vi "Scope1.vi"(2 "错误输入":errorcluster caption="错误输出") -> (0 "错误输出":errorcluster)   [LabVIEW 2012]
uses:
  Program Files (x86)/National Instruments/LabVIEW 2018/instr.lib/Tektronix DPO MSO 2000 4000 Series/Tektronix DPO MSO 2000 4000 Series.lvlib
panel:
  out "Busy":bool
  in  "电压范围":u64(ring)=10 items=["1 V"=1000000, "100mv"=100000, "10mv"=10000, "1mv"=1000, "100uv"=100, "10uv"=10]
  in  "时间范围":u64(ring)=100000 items=["100ms"=1000000000, "10ms"=100000000, "1ms"=10000000, "100us"=1000000, "10us"=100000, "1us"=10000, "100ns"=1000, "10ns"=100, "1ns"=10, "100ps"=1]
  in  "Channel":T1(ring)
  in  "停止":bool
  in  "开始测量":bool
  in  "更改参数":bool
  out "示波器通信":bool caption="通信正常"
  out "重频":dbl format="%.2f"
  out "脉宽":dbl format="%.2f"
  out "时间波形":waveform(dbl)(graph)
  # "时间波形"
  # "脉冲宽度"
  # "ns"
  # "重复频率"
  # "hz"
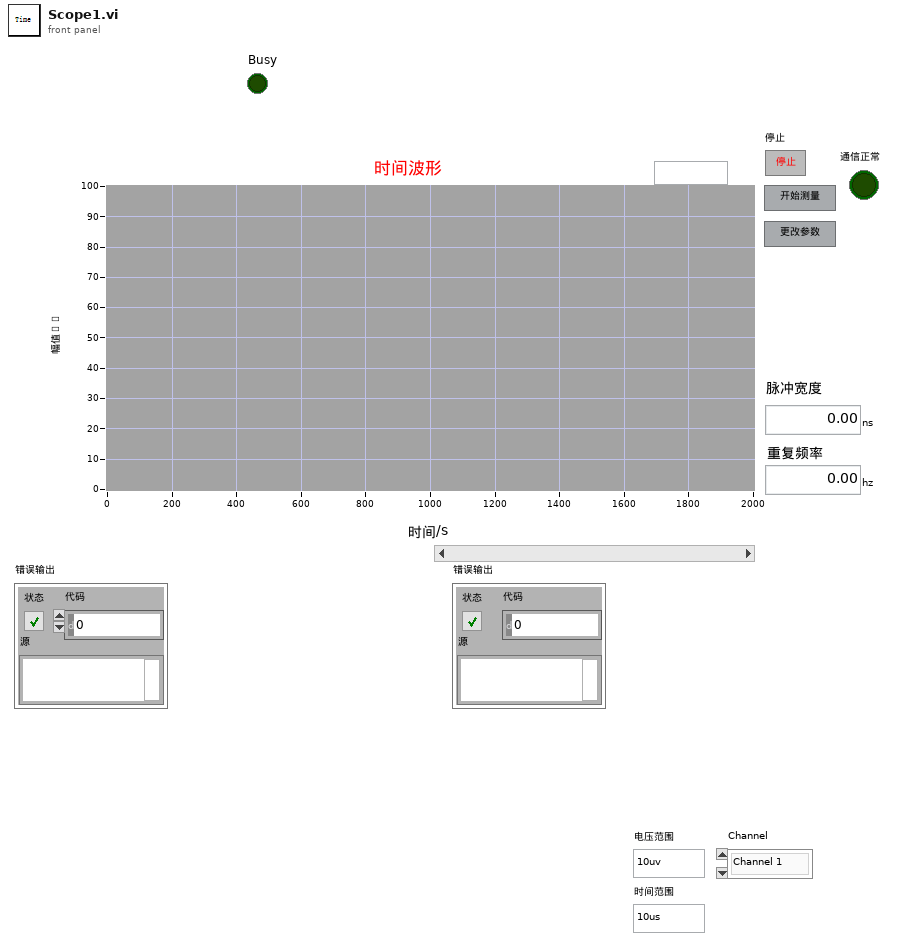
[diagram p1: front panel]
types:
  T1 = enum16{"Channel 1", "Channel 2", "Channel 3", "Channel 4"}
  T2 = typedef "IMAQ Image.ctl" = refnum<image>
  T3 = cluster{"示波器":cluster{"Channel (0:Channel 1)":enum16{"Channel 1", "Channel 2", "Channel 3", "Channel 4"}, "电压范围":dbl, "触发电压":dbl, "时间范围":dbl, " 示波器VISA":refnum<visa-resource-name>}, "光谱仪":cluster{"Channel (0:Channel 1)":enum16{"Channel 1", "Channel 2", "Channel 3", "Channel 4"}, "电压范围":u64, "触发电压":u64, "时间范围":u64}, " 相机1":cluster{"曝光时间":i32, "模拟增益":i32, "控制套接字":i32, "IP 地址":string, " 采集套接字":i32, "  版本号":i32, "ImageData":T2, "  增益最大":i32, "  增益最小":i32, " 曝光最大":i32, " 曝光最小":i32, " 帧速":i32, " 同步切换":i32, "  曝光缩放":i32}, " 偏振仪":cluster{"波长范围":enum16{"可见光", "近红外"}, "电压范围":u64, "触发电压":u64, "时间范围":u64}, " 功率计":cluster{"通道":enum16{"Channel 1", "Channel 2"}, "工作波长":u64, "单位":u64, "时间范围":u64}, "能量计":cluster{"通道":enum16{"Channel 1", "Channel 2"}, "工作波长":u64, "单位":u64, "时间范围":u64}, "电机":cluster{"Channel (0:Channel 1)":enum16{"Channel 1", "Channel 2", "Channel 3", "Channel 4"}, "电压范围":u64, "触发电压":u64, "时间范围":u64}}
  T4 = cluster{"Channel (0:Channel 1)":enum16{"Channel 1", "Channel 2", "Channel 3", "Channel 4"}, "电压范围":dbl, "触发电压":dbl, "时间范围":dbl, " 示波器VISA":refnum<visa-resource-name>}
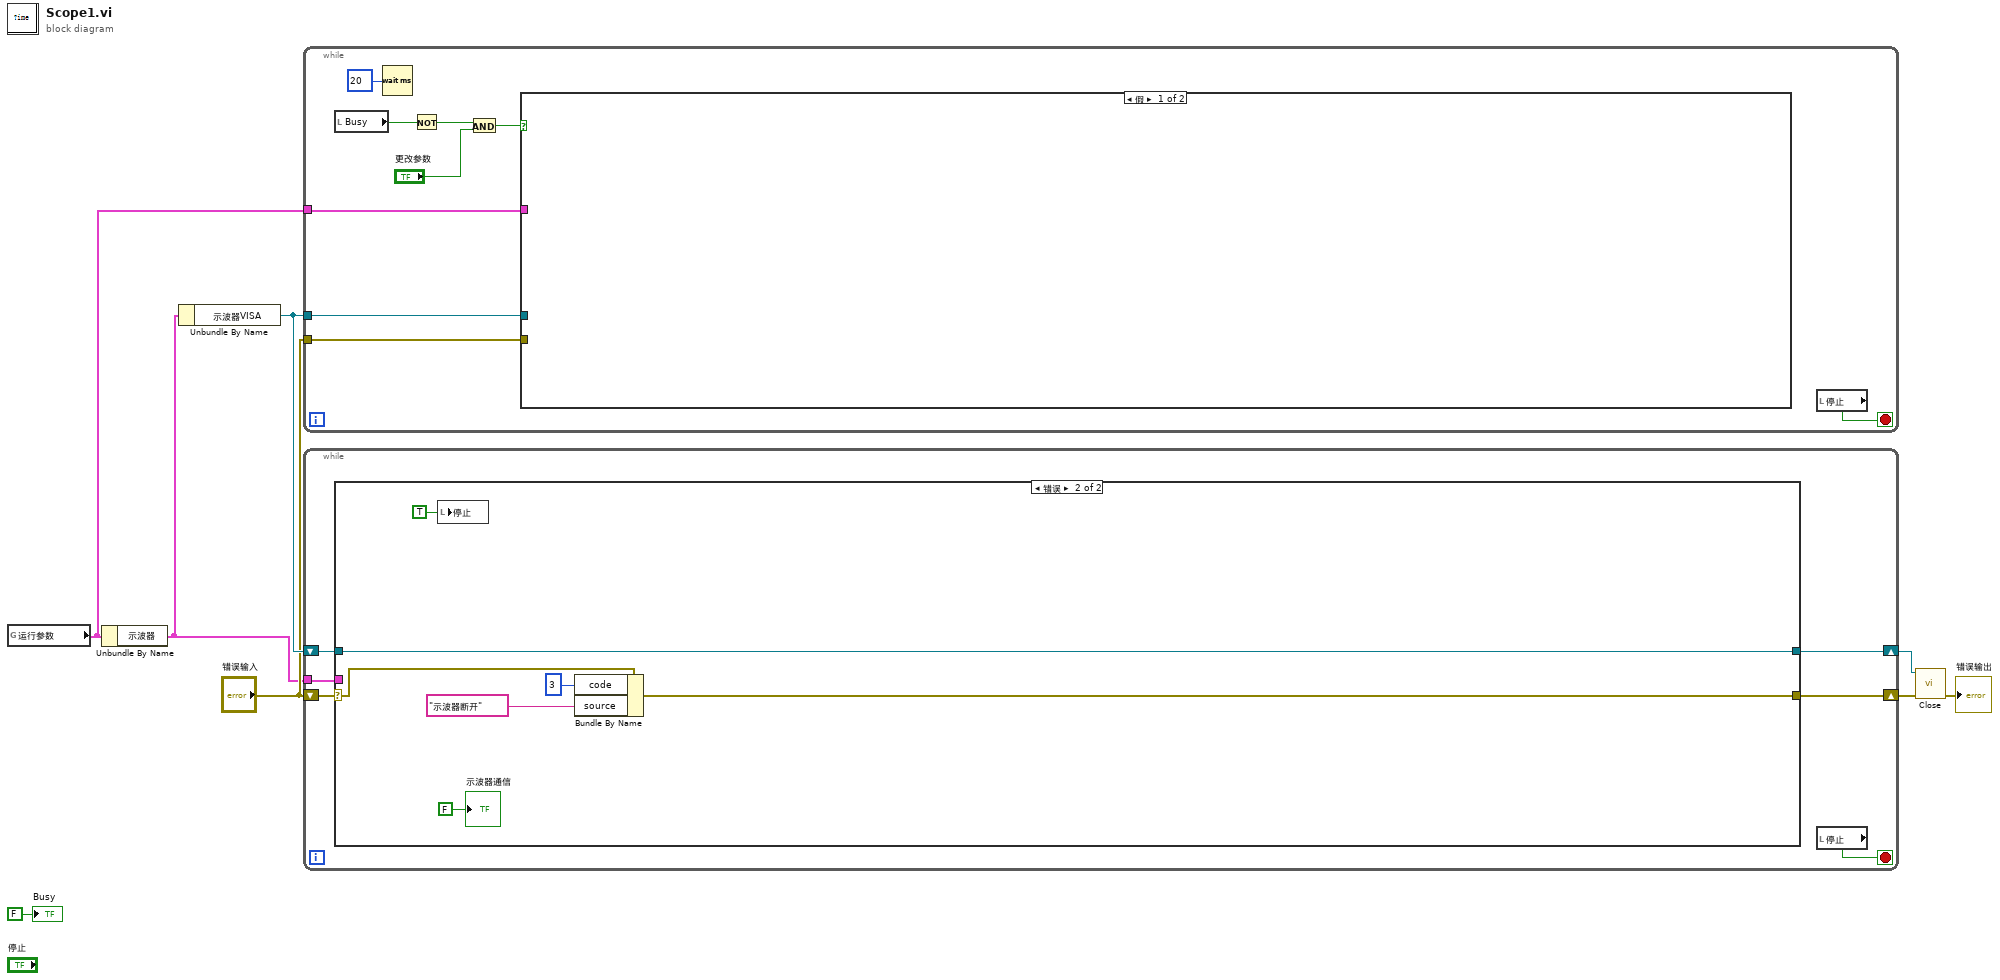
[diagram p0: block diagram]
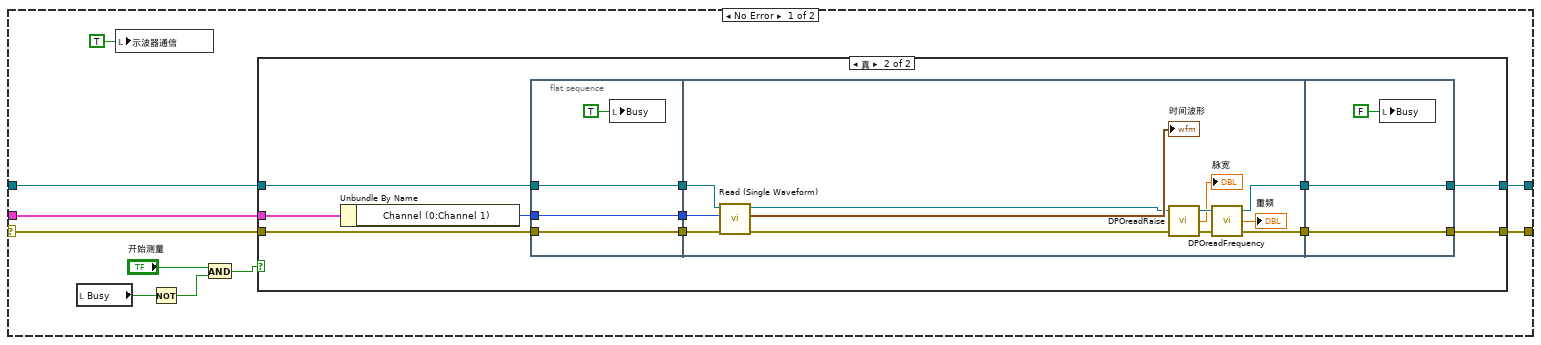
[diagram p2: hidden frame]
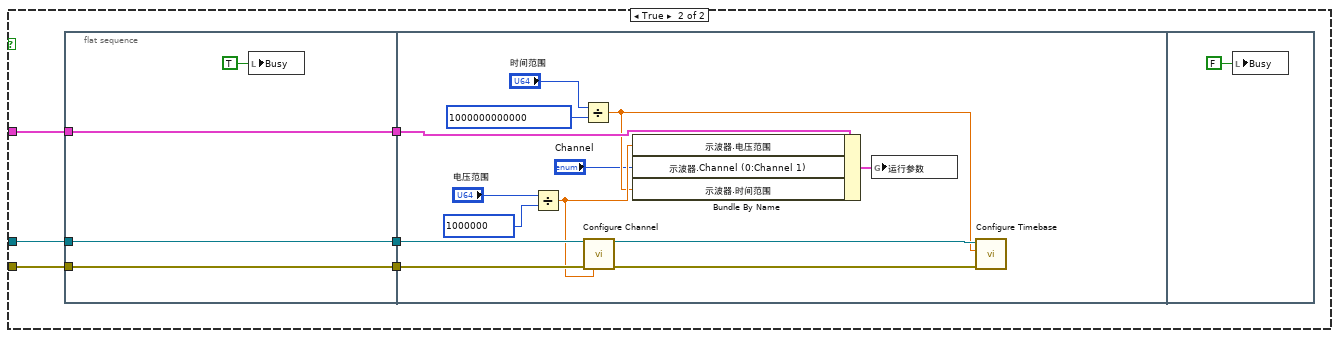
[diagram p4: hidden frame]
diagram:
  n1 = global read "参数.vi" "运行参数"() -> (w4:T3)
  n2 = Unbundle By Name(w4) -> ("示波器"=w1:T4)
  n3 = Unbundle By Name(w1) -> ("示波器VISA"=w5:refnum<visa-resource-name>)
  n4 = while {
    tunnel: w5 -> [w16]
    tunnel: w4 -> [w15]
    tunnel: "错误输入" -> [w14]
    stop <- w17 stop-if-true
    n5 = local read "Busy"() -> (w13:bool)
    n6 = Wait (ms)(milliseconds to wait=u32 20 ("等待时间（毫秒）")) -> ()  [unwired: 1 out]
    n7 = Not(x=w13) -> (.not. x?=w12:bool)
    n8 = And(x=w12, y="更改参数") -> (x .and. y?=w10:bool)
    n9 = case shown="假" w10 {
      tunnel: w16 -> [_ w23]
      tunnel: w15 -> [_ w22]
      tunnel: w14 -> [_ w21]
      frame False {
      }
      frame True {
        n10 = flat-sequence {
          tunnel: w21 -> [w25]
          tunnel: w22 -> [w26]
          tunnel: w23 -> [w27]
          tunnel: [w27] -> w20
          tunnel: [w26] -> w19
          tunnel: [w25] -> w18
          tunnel: w20 -> [w40]
          tunnel: w19 -> [w39]
          tunnel: w18 -> [w38]
          frame #0 {
            n11 = local write "Busy"(TRUE ("Busy")) -> ()
          }
          frame #1 {
            n12 = Divide(x="电压范围", y=u64 1000000) -> (x/y=w31:dbl)
            n13 = Divide(x="时间范围", y=u64 1000000000000) -> (x/y=w30:dbl)
            n14 = call "Configure Channel.vi"("VISA resource name"=w40, "error in (no error)"=w38, "Vertical Range (10.0 V)"=w31) -> ("VISA resource name out"=w33:refnum<visa-resource-name>, "error out"=w32:errorcluster)  [unwired: 11 in]
            n15 = Bundle By Name(cluster=w39, "示波器.电压范围"=w31, "示波器.Channel (0:Channel 1)"="Channel", "示波器.时间范围"=w30) -> (w28:T3)
            n16 = global write "参数.vi" "运行参数"(w28) -> ()
            n17 = call "Configure Timebase.vi"("error in (no error)"=w32, "Timebase (0.0005 s)"=w30, "VISA resource name"=w33) -> ()  [unwired: 7 in, 2 out]
          }
          frame #2 {
            n18 = local write "Busy"(FALSE ("Busy")) -> ()
          }
        }
      }
    }
    n19 = local read "停止"() -> (w17:bool)
  }
  n20 = while {
    shift-right: [w47] -> w8
    shift-left: w5 -> [w45]
    shift-right: [w46] -> w7
    shift-left: "错误输入" -> [w43]
    tunnel: w1 -> [w44]
    stop <- w42 stop-if-true
    n21 = case shown="错误" w43 {
      selector: w43 -> [w48 w94]
      tunnel: [w57 w95] -> w47
      tunnel: [w56 w91] -> w46
      tunnel: w45 -> [w55 w95]
      tunnel: w44 -> [w53 _]
      frame No Error {
        n22 = local read "Busy"() -> (w51:bool)
        n23 = local write "示波器通信"(TRUE ("示波器通信")) -> ()
        n24 = Not(x=w51) -> (.not. x?=w50:bool)
        n25 = And(x="开始测量", y=w50) -> (x .and. y?=w49:bool)
        n26 = case shown="真" w49 {
          tunnel: w55 -> [w59 w68]
          tunnel: [w59 w70] -> w57
          tunnel: [w58 w69] -> w56
          tunnel: w48 -> [w58 w67]
          tunnel: w53 -> [_ w66]
          frame False {
          }
          frame True {
            n27 = Unbundle By Name(w66) -> ("Channel (0:Channel 1)"=w65:T1)
            n28 = flat-sequence {
              tunnel: w65 -> [w72]
              tunnel: w67 -> [w73]
              tunnel: w68 -> [w74]
              tunnel: [w74] -> w62
              tunnel: [w73] -> w61
              tunnel: [w72] -> w60
              tunnel: [w79] -> w64
              tunnel: [w78] -> w63
              tunnel: w62 -> [w77]
              tunnel: w61 -> [w76]
              tunnel: w60 -> [w75]
              tunnel: [w88] -> w69
              tunnel: [w89] -> w70
              tunnel: w64 -> [w89]
              tunnel: w63 -> [w88]
              frame #0 {
                n29 = local write "Busy"(TRUE ("Busy")) -> ()
              }
              frame #1 {
                n30 = call "Read (Single Waveform).vi"("error in (no error)"=w76, "Channel (0: Channel 1)"=w75, "VISA resource name"=w77) -> ("error out"=w84:errorcluster, "Waveform Graph"=→"时间波形":waveform(dbl), "VISA resource name out"=w85:refnum<visa-resource-name>)  [unwired: 6 in]
                n31 = call "DPOreadRaise.vi"("错误输入（无错误）"=w84, "VISA资源名称"=w85) -> ("错误输出"=w82:errorcluster, "上升沿时间"=→"脉宽":dbl, "VISA资源名称输出"=w83:refnum<visa-resource-name>)  [unwired: 1 in]
                n32 = call "DPOreadFrequency.vi"("错误输入（无错误）"=w82, "VISA资源名称"=w83) -> ("错误输出"=w78:errorcluster, "重复频率"=→"重频":dbl, "VISA资源名称输出"=w79:refnum<visa-resource-name>)  [unwired: 1 in]
              }
              frame #2 {
                n33 = local write "Busy"(FALSE ("Busy")) -> ()
              }
            }
          }
        }
      }
      frame Error {
        n34 = local write "停止"(TRUE) -> ()
        n35 = Bundle By Name(cluster=w94, "code"=3, "source"="示波器断开") -> (w91:errorcluster)
        "示波器通信" <- FALSE
      }
    }
    n36 = local read "停止"() -> (w42:bool)
  }
  n37 = call "Close.vi"("error in (no error)"=w7, "VISA resource name"=w8) -> ("error out"=→"错误输出":errorcluster)  [unwired: 9 in]
  "Busy" <- FALSE ("Busy")
